vi "main_LAPD_display_voltage.vi"() -> ()   [LabVIEW 2009]
panel:
  in  "Stopp":bool
  in  "LAPD-Kanal an Meilhauskarte":u32 max=31
  out "LAPD Spannung (V)":dbl
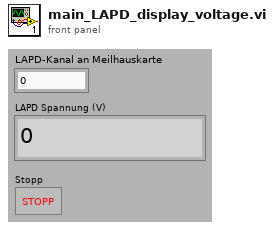
[diagram p1: front panel]
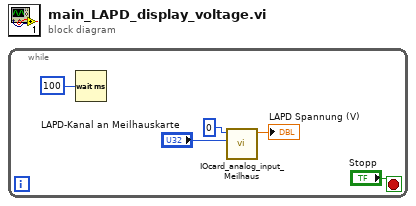
[diagram p0: block diagram]
diagram:
  n1 = while {
    stop <- "Stopp" stop-if-true
    n2 = Wait (ms)(milliseconds to wait=u32 100 ("Zu wartende ms")) -> ()  [unwired: 1 out]
    n3 = call "IOcard_analog_input_Meilhaus.vi"("Channel"="LAPD-Kanal an Meilhauskarte", "Device"=u32 0 ("Board Number")) -> ("Voltage [V]"=→"LAPD Spannung (V)":dbl)  [unwired: 9 in]
  }
